vi "Test - Merge JSON - Array.vi"   [LabVIEW 2020, in "JSON Schema Generator.lvlib"]
uses:
  JSON Schema Generator.lvlib
  <vilib>/addons/_JKI Toolkits/Caraya/classes/Test/Test.lvclass
  <vilib>/addons/_JKI Toolkits/Caraya/classes/Assert/Assert.lvclass
  <vilib>/addons/_JKI Toolkits/Caraya/classes/Assert/Assert Not Error.vi
  <vilib>/addons/_JKI Toolkits/Caraya/classes/Assert/Assert Equal Value_Variant.vi
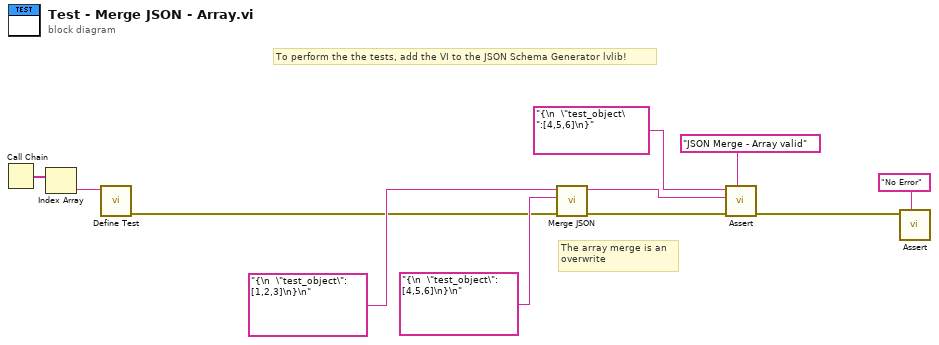
[diagram p0: block diagram]
diagram:
  # "To perform the the tests, add the VI to the JSON Schema Generator lvlib!"
  # "The array merge is an \noverwrite"
  n1 = Call Chain() -> (call chain=w9:string[])
  n2 = Index Array(array=w9) -> (element=w8:string)  [unwired: 1 in]
  n3 = call <vilib>:"Define Test.vi"("Label (VI Title)"=w8) -> ("error out"=w4:errorcluster)  [unwired: 9 in, 1 out]
  n4 = call "Merge JSON.vi"("error in (no error)"=w4, "<JSON> to merge in"="{\n  \"test_object\": [4,5,6]\n}\n", "<JSON> in"="{\n  \"test_object\": [1,2,3]\n}\n") -> ("error out"=w1:errorcluster, "<JSON> out"=w3:string)  [unwired: 7 in]
  n5 = call-poly <vilib>:"Assert.vi"("Label"="JSON Merge - Array valid", "error in (no error)"=w1, "Actual"=w3, "Expected"="{\n  \"test_object\":[4,5,6]\n}" ("<JSON> in")) -> ("error out"=w6:errorcluster)  [unwired: 6 in, 1 out]
  n6 = call-poly <vilib>:"Assert.vi"("Label"="No Error", "Not Error?"=w6) -> ()  [unwired: 8 in, 2 out]
